vi "Configure Runt Trigger.vi"(0 "VISA resource name":refnum<visa-resource-name>, 1 "Trigger Slope (0: Rising)":u16(ring) items=["Rising", "Falling"], 2 "Trigger Source (0: Channel 1)":u16(ring) items=["Channel 1", "Channel 2", "Channel 3", "Channel 4", "External", "Ext", "Ext10"], 5 "Lower Level (0.0 V)":dbl, 7 "Upper Level (0.0 V)":dbl, 9 "Mode (0: Less Than)":u16(ring) items=["Less Than", "Greater Than", "In Range / Out of Range"], 11 "error in (no error)":errorcluster, 12 "Limit 1 (4 ns)":dbl=4e-09, 13 "Limit 2 (6 ns)":dbl=6e-09) -> (4 "VISA resource name out":refnum<visa-resource-name>, 15 "error out":errorcluster)   [LabVIEW 2018, in "LeCroy Wave Series.lvlib"]
doc: "Configures runt trigger settings. The runt trigger is programmed to occur when a pulse crosses a first threshold line and fails to cross a second threshold line before recrossing the first.\n\nNotes:\n 1) \"External\" is included for the purpose of backwards compatibility. Use EXT or EXT10 for best results.\n\n2) This trigger type is not supported on all scopes."
uses:
  LeCroy Wave Series.lvlib
panel:
  # "Note: \"External\" is included for the purposeof backwards compatibility.  Use EXT or EXT10for best results."
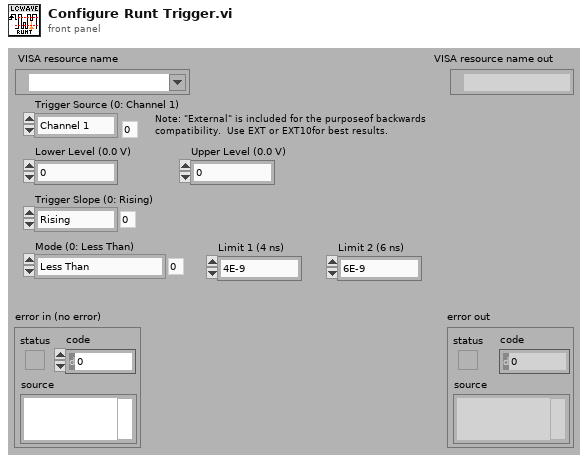
[diagram p1: front panel]
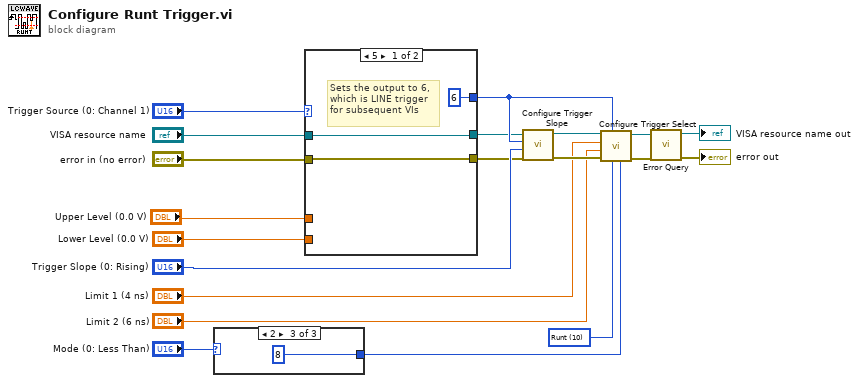
[diagram p0: block diagram]
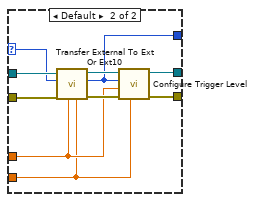
[diagram p2: hidden frame]
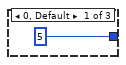
[diagram p3: hidden frame]
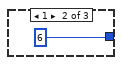
[diagram p4: hidden frame]
diagram:
  w7 = u16 10 items=["Edge", "Dropout", "Glitch", "Interval", "Std", "Sng", "State Qualify", "Edge Qualify", "Width", "Logic", "Runt"] ("Trigger type")
  n1 = case shown="2" "Mode (0: Less Than)" {
    tunnel: [5 6 8] -> w15
    frame 0, Default {
    }
    frame 1 {
    }
    frame 2 {
    }
  }
  n2 = case shown="5" "Trigger Source (0: Channel 1)" {
    selector: "Trigger Source (0: Channel 1)" -> [_ w27]
    tunnel: "VISA resource name" -> [w25 w36]
    tunnel: "error in (no error)" -> [w24 w35]
    tunnel: [u16 6 ("Trigger Source With Ext/Ext10") w32] -> w6
    tunnel: [w24 w31] -> w5
    tunnel: [w25 w30] -> w4
    tunnel: "Upper Level (0.0 V)" -> [_ w29]
    tunnel: "Lower Level (0.0 V)" -> [_ w28]
    frame 5 {
      # "Sets the output to 6,\nwhich is LINE trigger\nfor subsequent VIs"
    }
    frame Default {
      n3 = call "Transfer External To Ext Or Ext10.vi"("Trigger Level 2"=w28, "Trigger Level"=w29, "error in (no error)"=w35, "Trigger Source With External"=w27, "VISA resource name"=w36) -> ("error out"=w33:errorcluster, "Trigger Source With Ext/Ext10"=w32:u16, "VISA resource name out"=w34:refnum<visa-resource-name>)  [unwired: 4 in]
      n4 = call "Configure Trigger Level.vi"("Trigger Level 2 (0.0 V)"=w28, "error in (no error)"=w33, "Trigger Level 1 (0.0 V)"=w29, "Channel (0: Channel 1)"=w32, "VISA resource name"=w34) -> ("error out"=w31:errorcluster, "VISA resource name out"=w30:refnum<visa-resource-name>)  [unwired: 5 in]
    }
  }
  n5 = call "Configure Trigger Slope.vi"("error in (no error)"=w5, "Trigger Slope (0: Rising)"="Trigger Slope (0: Rising)", "Channel (0: Channel 1)"=w6, "VISA resource name"=w4) -> ("error out"=w19:errorcluster, "VISA resource name out"=w20:refnum<visa-resource-name>)  [unwired: 6 in]
  n6 = call "Configure Trigger Select.vi"("Hold Type (0: TI)"=w15, "Trigger type"=w7, "Trigger Source (0: Channel 1)"=w6, "error in (no error)"=w19, "Hold Value 2 (6 ns)"="Limit 2 (6 ns)", "Hold Value 1 (4 ns)"="Limit 1 (4 ns)", "VISA resource name"=w20) -> ("error out"=w10:errorcluster, "VISA resource name out"=w11:refnum<visa-resource-name>)  [unwired: 3 in]
  n7 = call "Error Query.vi"("error in (no error)"=w10, "VISA resource name"=w11) -> ("error out"=→"error out":errorcluster, "VISA resource name out"=→"VISA resource name out":refnum<visa-resource-name>)  [unwired: 6 in, 2 out]
